vi "Smartwatch - .vi"() -> ()   [LabVIEW 2025]
uses:
  <vilib>/Utility/miscctls.llb/LVPoint32TypeDef.ctl
  <vilib>/Instr/_visa.llb/VISA Configure Serial Port (Instr).vi
panel:
  out "Timer Status":bool
  in  "Smartwatch Display":enum32{"Ekran g³ówny", "Krokomierz", "Stoper"}(tab)
  out "Time Dispay":string
  out "Liczba Kroków (bieg)":i32
  out "Liczba Kroków":i32
  out "Waveform Chart [Magnitude]":cluster{dbl, dbl, dbl}(graph)
  out "Status":string
  in  "STOP Button":bool
  out "Status":bool
  in  "START Button":bool
  in  "Timer START":bool
  in  "Timer STOP":bool
  out "Timer value":u32
  out "Waveform Chart [X+Y+Z]":cluster{dbl, dbl, dbl}(graph)
  out "x*y 3":dbl
  out "x*y 2":dbl
  out "x*y 1":dbl
  out "Smartwatch":picture
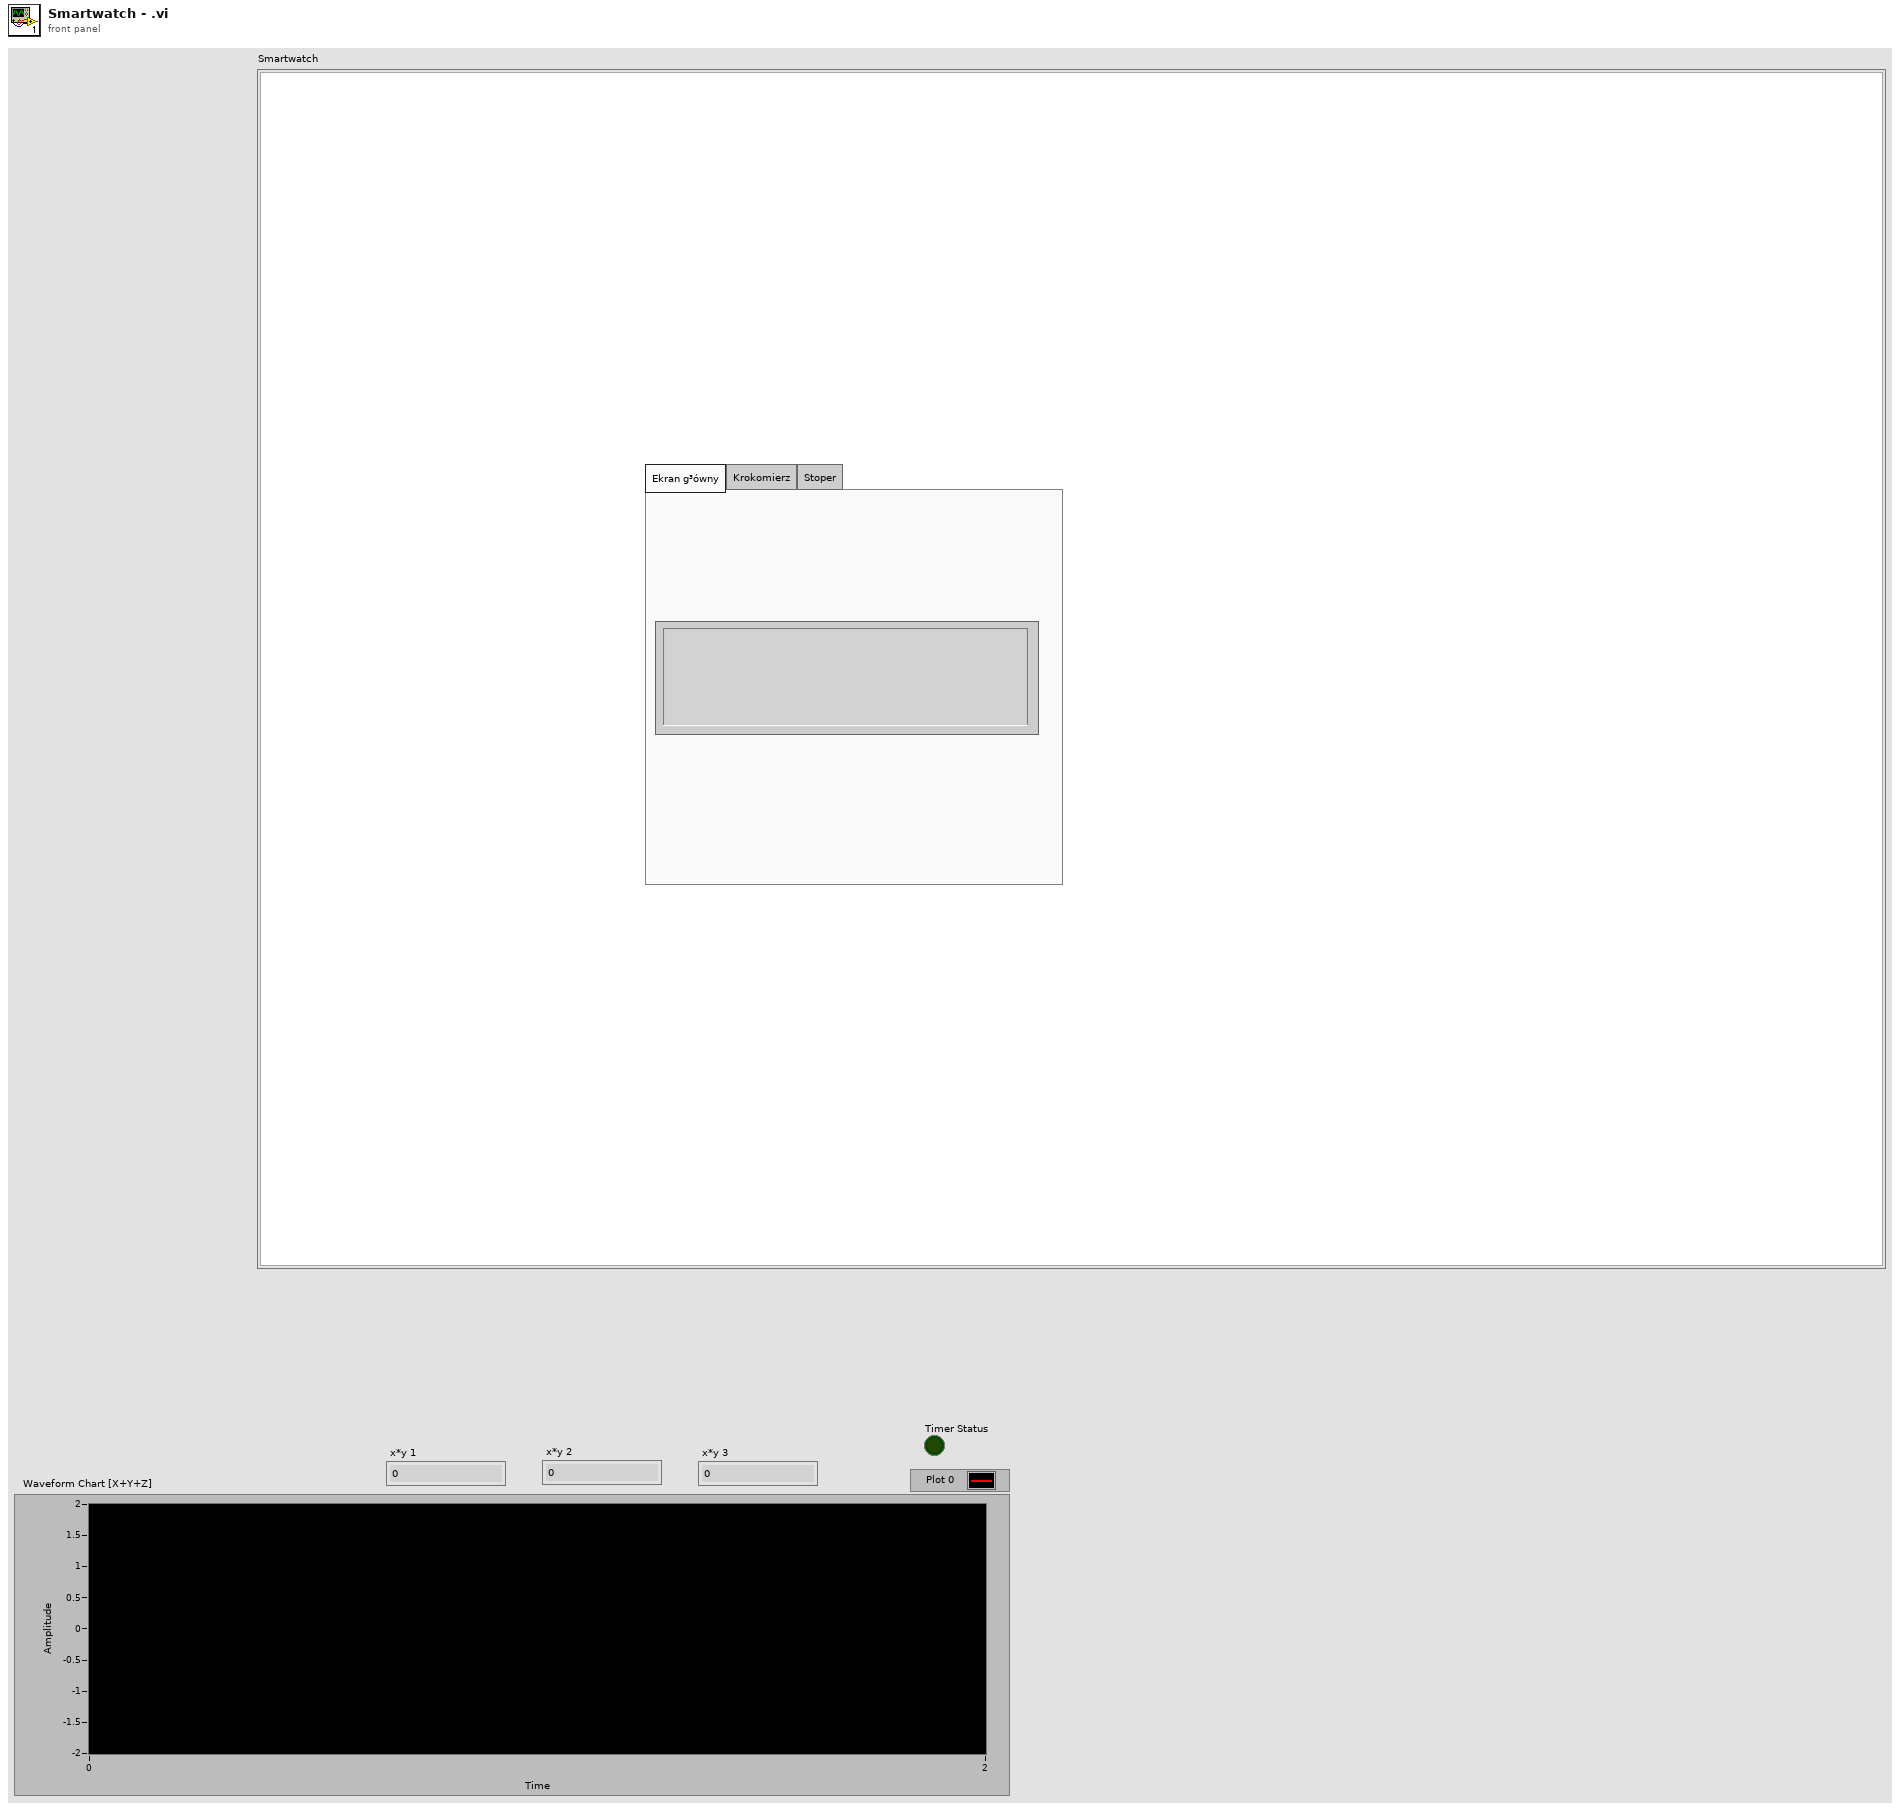
[diagram p1: front panel]
types:
  T1 = typedef "LVPoint32TypeDef.ctl" = cluster{"Horizontal":i32, "Vertical":i32}
  T2 = typedef "imagedata.ctl" = cluster{"image type":i32, "image depth":i32, "image":u8[], "mask":u8[], "colors":u32[], "Rectangle":cluster{"left":i16, "top":i16, "right":i16, "bottom":i16}}
  T3 = cluster{"Acceleration [g] -2.0<->+2.0 ":dbl, "Acceleration [g] -2.0<->+2.0 ":dbl, "Acceleration [g] -2.0<->+2.0 ":dbl}
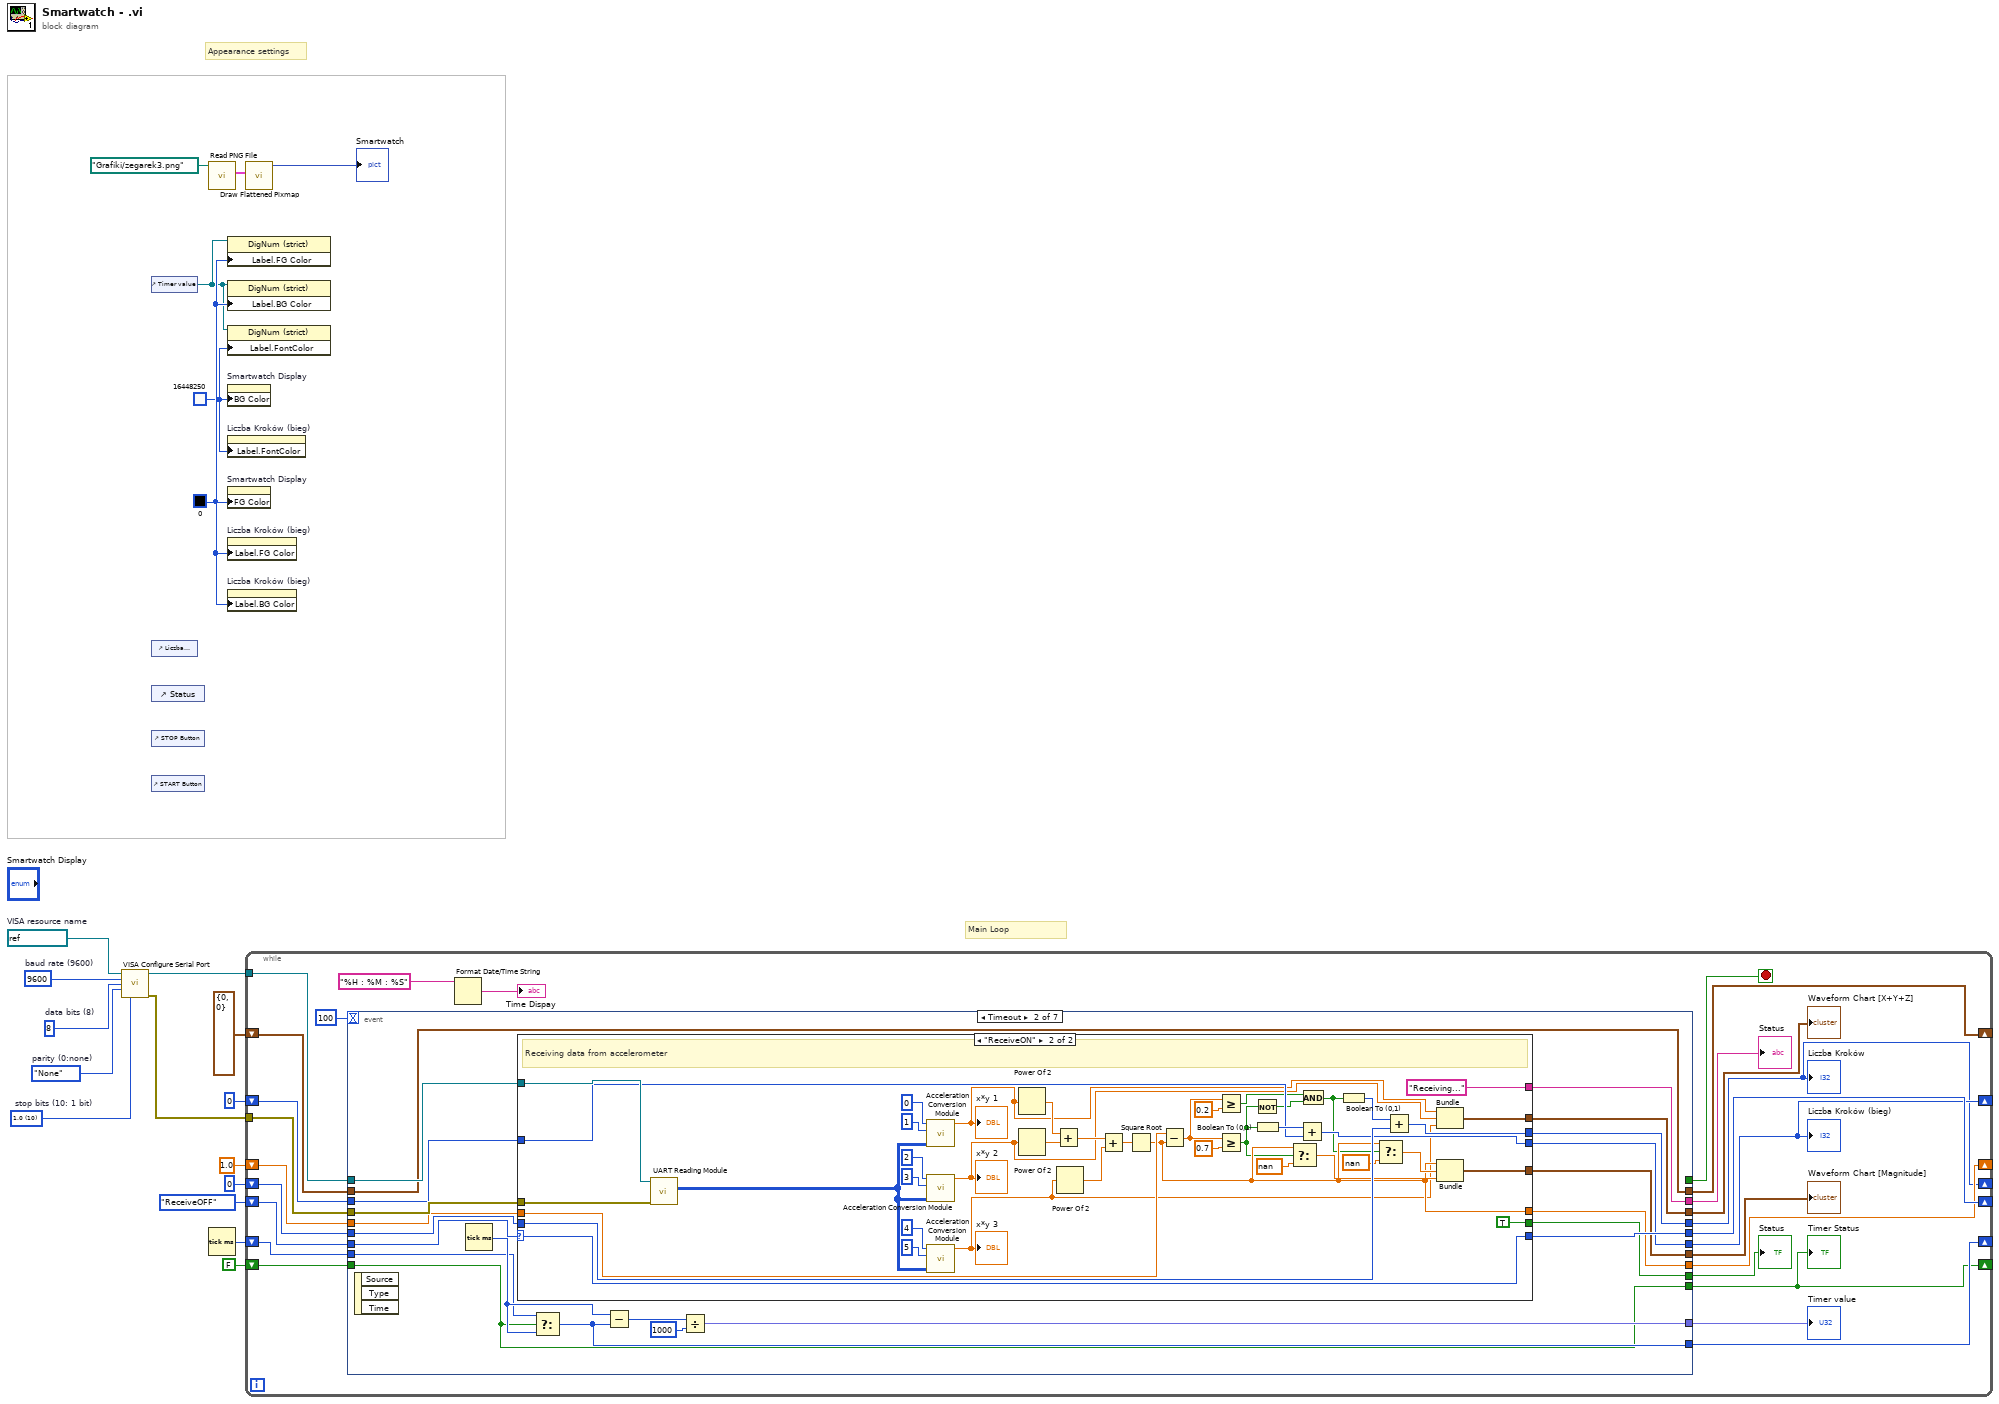
[diagram p0: block diagram]
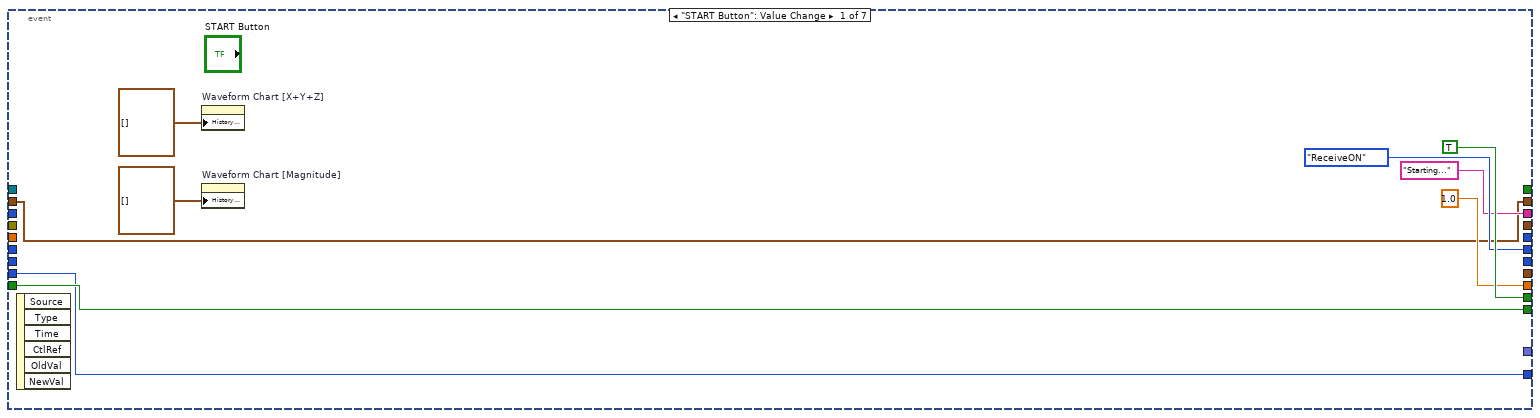
[diagram p2: hidden frame]
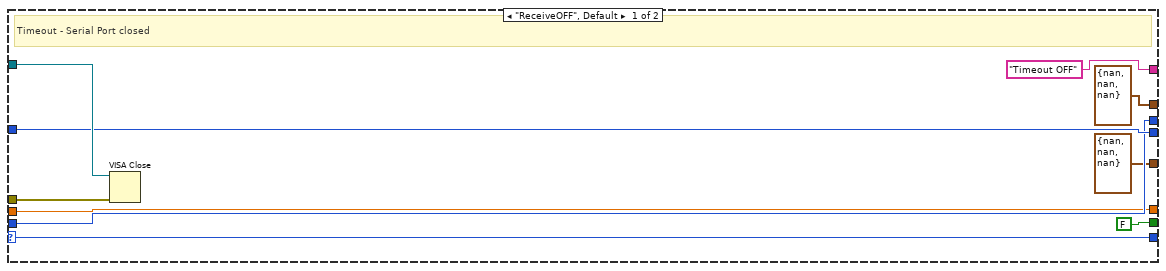
[diagram p3: hidden frame]
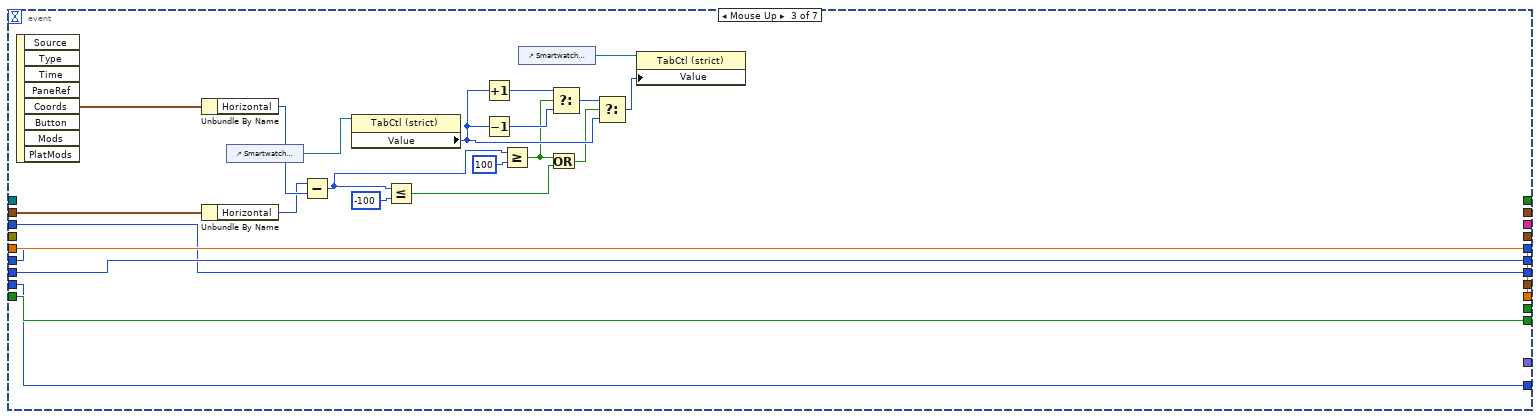
[diagram p4: hidden frame]
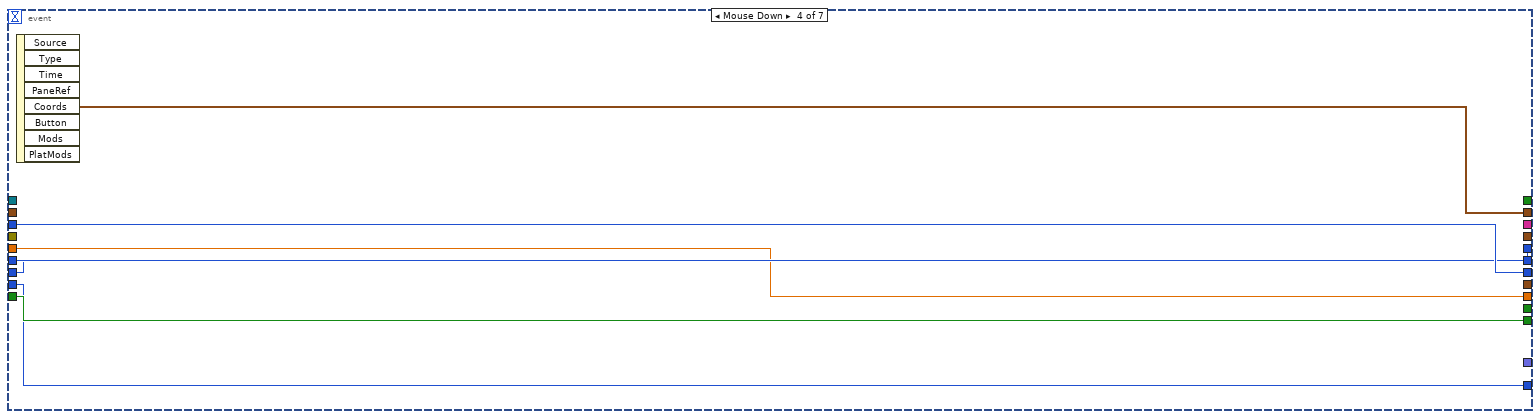
[diagram p5: hidden frame]
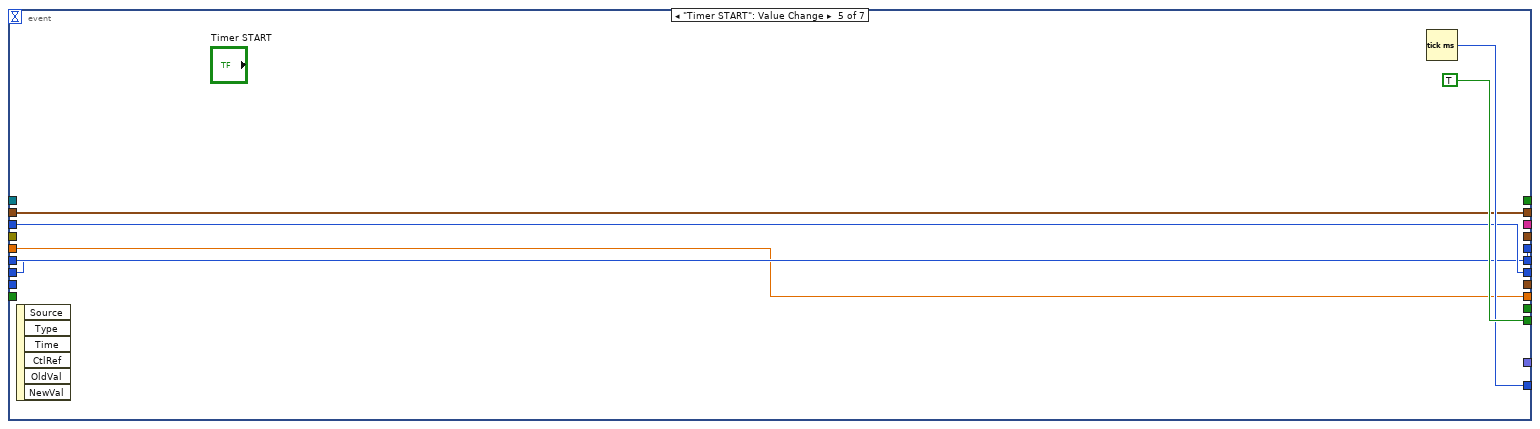
[diagram p6: hidden frame]
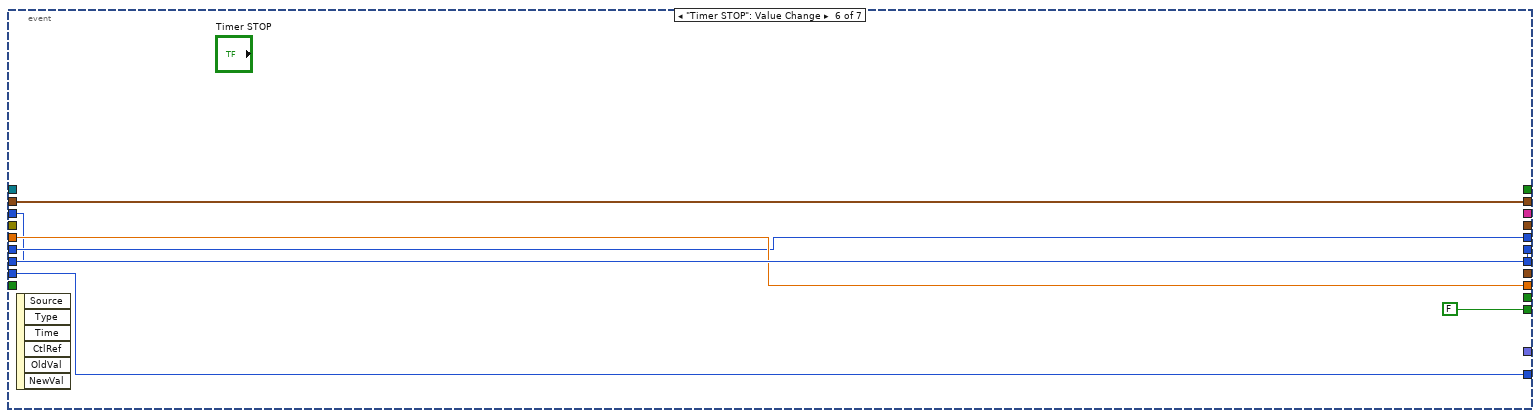
[diagram p7: hidden frame]
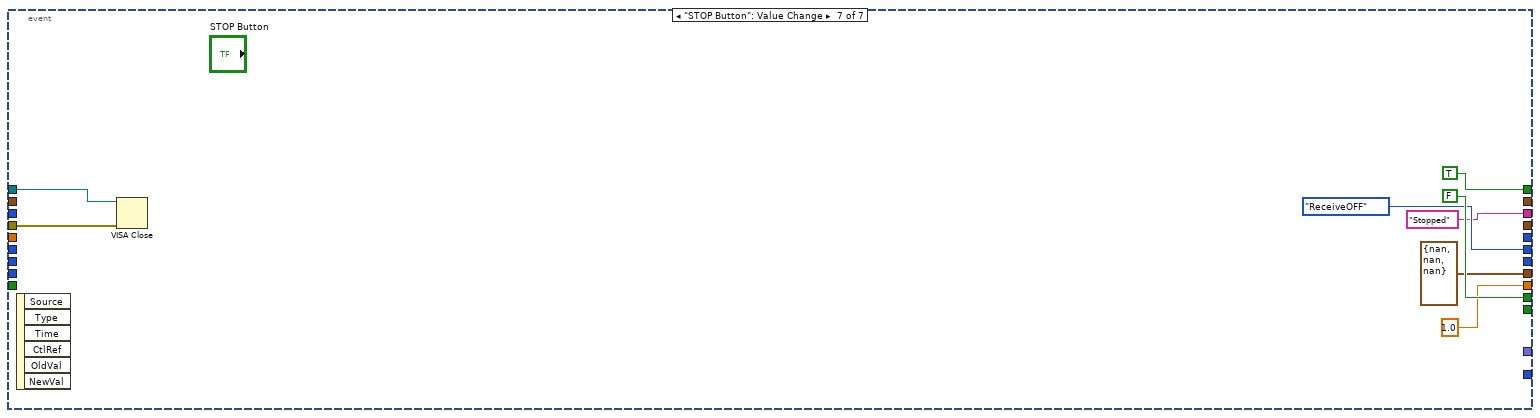
[diagram p8: hidden frame]
diagram:
  w5 = u32 16448250 ("Colors:BG Color")
  w6 = u32 0 ("Colors:BG Color")
  w14 = enum16{"None", "Odd", "Even", "Mark", "Space"}."None"  # parity (0:none)
  w15 = u16 8  # data bits (8)
  w16 = u16 10 items=["1.0"=10, "1.5"=15, "2.0"=20]  # stop bits (10: 1 bit)
  w17 = u32 9600  # baud rate (9600)
  w18 = refnum<visa-resource-name> "COM3"  # VISA resource name
  # "Main Loop"
  # "Appearance settings"
  n1 = call-poly "VISA Configure Serial Port"("VISA resource name"=w18, "baud rate (9600)"=w17, "data bits (8)"=w15, "parity (0:none)"=w14, "stop bits (10: 1 bit)"=w16) -> ("VISA resource name out"=w20:refnum<visa-resource-name>, "error out"=w19:errorcluster)  [unwired: 9 in]
  n2 = control-ref of="Timer value"() -> (w4:refnum<vi>)
  n3 = control-ref of="Liczba Kroków"() -> ()  [unwired: 1 out]
  n4 = control-ref of="Status"() -> ()  [unwired: 1 out]
  n5 = control-ref of="STOP Button"() -> ()  [unwired: 1 out]
  n6 = control-ref of="START Button"() -> ()  [unwired: 1 out]
  n7 = call <vilib>:"Read PNG File.vi"("path to PNG file"=path "Grafiki/zegarek3.png") -> ("image data"=w8:T2)  [unwired: 8 in, 2 out]
  n8 = Tick Count (ms)() -> (millisecond timer value=w3:u32)
  n9 = property on="Property Node" class="DigNum (strict)"(reference=w4, "Label.FG Color"=w6) -> ()  [unwired: 1 in, 2 out]
  n10 = property on="Property Node" class="DigNum (strict)"(reference=w4, "Label.BG Color"=w6) -> ()  [unwired: 1 in, 2 out]
  n11 = property on="Property Node" class="DigNum (strict)"(reference=w4, "Label.FontColor"=w5) -> ()  [unwired: 1 in, 2 out]
  n12 = property on="Smartwatch Display" class="TabCtl (strict)"("BG Color"=w5) -> ()  [unwired: 2 in, 2 out]
  n13 = property on="Liczba Kroków (bieg)" class="DigNum (strict)"("Label.FontColor"=w5) -> ()  [unwired: 2 in, 2 out]
  n14 = property on="Smartwatch Display" class="TabCtl (strict)"("FG Color"=w6) -> ()  [unwired: 2 in, 2 out]
  n15 = property on="Liczba Kroków (bieg)" class="DigNum (strict)"("Label.FG Color"=w6) -> ()  [unwired: 2 in, 2 out]
  n16 = property on="Liczba Kroków (bieg)" class="DigNum (strict)"("Label.BG Color"=w6) -> ()  [unwired: 2 in, 2 out]
  n17 = call <vilib>:"Draw Flattened Pixmap.vi"("image data"=w8) -> ("new picture"=→"Smartwatch":picture)  [unwired: 8 in]
  n18 = while {
    tunnel: w19 -> [w44]
    tunnel: w20 -> [w45]
    shift-right: [w40] -> _
    shift-left: enum16{"ReceiveOFF", "ReceiveON"}."ReceiveOFF" -> [w41]
    shift-right: [w37] -> _
    shift-left: 1.0 -> [w36]
    shift-right: [w32] -> _
    shift-left: 0 -> [w35]
    shift-right: [w33] -> _
    shift-left: 0 -> [w34]
    shift-right: [w29] -> _
    shift-left: w3 -> [w25]
    shift-right: [w26] -> _
    shift-left: FALSE -> [w28]
    shift-right: [w23] -> _
    shift-left: T1 {"Horizontal"=0, "Vertical"=0} ("Coords") -> [w24]
    stop <- w42 stop-if-true
    n19 = event shown="[1] Timeout" {
      selector: _ -> [_ _ _ _ _ _ _]
      dyn-events: _ -> [_ _ _ _ _ _ _]
      timeout: 100 -> [_ _ _ _ _ _ _]
      tunnel: w45 -> [_ w74 _ _ _ _ w179]
      tunnel: w44 -> [_ w73 _ _ _ _ w178]
      tunnel: [TRUE w72 _ _ _ _ FALSE] -> w43
      tunnel: [_ _ _ _ _ _ TRUE] -> w42
      tunnel: w41 -> [_ w76 w133 w153 w159 w168 _]
      tunnel: [enum16{"ReceiveOFF", "ReceiveON"}."ReceiveON" w75 w133 w153 w159 w168 enum16{"ReceiveOFF", "ReceiveON"}."ReceiveOFF"] -> w40
      tunnel: ["Starting..." ("Status") w71 _ _ _ _ "Stopped" ("Status")] -> w38
      tunnel: [1.0 ("Magnitude Old") w70 w132 w154 w160 w167 1.0] -> w37
      tunnel: w36 -> [_ w69 w132 w154 w160 w167 _]
      tunnel: w35 -> [_ w68 w130 w155 w161 w166 _]
      tunnel: w34 -> [_ w67 w131 w156 w162 w165 _]
      tunnel: [_ w66 w130 w155 w161 w166 _] -> w32
      tunnel: [_ w65 w131 w156 w162 w165 _] -> w33
      tunnel: [_ w64 _ _ _ _ cluster{dbl, dbl, dbl} {nan, nan, nan}] -> w31
      tunnel: [_ w63 _ _ _ _ _] -> w30
      tunnel: w28 -> [w47 w56 w129 w152 _ _ _]
      tunnel: w25 -> [w46 w60 w128 w151 _ w169 _]
      tunnel: [w46 w58 w128 w151 w163 w169 _] -> w29
      tunnel: [_ w57 _ _ _ _ _] -> w27
      tunnel: [w47 w56 w129 w152 TRUE FALSE _] -> w26
      tunnel: w24 -> [w48 w55 w136 _ w158 w170 _]
      tunnel: [w48 w55 _ w157 w158 w170 _] -> w23
      event "START Button": Value Change {
        n20 = event-data() -> ()  [unwired: 1 in, 6 out]
        n21 = property on="Waveform Chart [X+Y+Z]" class="WFChart (strict)"("History Data"=cluster{dbl, dbl, dbl}[] []) -> ()  [unwired: 2 in, 2 out]
        n22 = property on="Waveform Chart [Magnitude]" class="WFChart (strict)"("History Data"=cluster{dbl, dbl, dbl}[] []) -> ()  [unwired: 2 in, 2 out]
      }
      event Timeout {
        n23 = event-data() -> ()  [unwired: 1 in, 3 out]
        n24 = Tick Count (ms)() -> (millisecond timer value=w62:u32)
        n25 = case shown="\"ReceiveON\"" w76 {
          selector: w76 -> [w78 w99]
          tunnel: [w78 w99] -> w75
          tunnel: w74 -> [w86 w127]
          tunnel: w73 -> [w85 w126]
          tunnel: [FALSE TRUE] -> w72
          tunnel: ["Timeout OFF" ("Status") "Receiving..." ("Status")] -> w71
          tunnel: [w80 w98] -> w70
          tunnel: w69 -> [w80 w114]
          tunnel: w68 -> [w81 w108]
          tunnel: w67 -> [w82 w109]
          tunnel: [w81 w106] -> w66
          tunnel: [w82 w105] -> w65
          tunnel: [cluster{dbl, dbl, dbl} {nan, nan, nan} w100] -> w64
          tunnel: [cluster{dbl, dbl, dbl} {nan, nan, nan} w90] -> w63
          frame "ReceiveOFF", Default {
            # "Timeout - Serial Port closed"
            n26 = VISA Close(VISA resource name=w86, error in (no error)=w85) -> ()  [unwired: 1 out]
          }
          frame "ReceiveON" {
            # "Receiving data from accelerometer"
            n27 = call "UART Reading Module.vi"("error in (no error)"=w126, "VISA Refnum in"=w127) -> ("Array with 6 col"=w121:u8[][])  [unwired: 7 in, 2 out]
            n28 = call "Acceleration Conversion Module.vi"("Array Input (1 row 6 col)"=w121, "Second column"=1, "First column"=0) -> ("Acceleration [g] -2.0<->+2.0"=w89:dbl)  [unwired: 6 in]
            "x*y 1" <- w89
            n29 = call "Acceleration Conversion Module.vi"("Array Input (1 row 6 col)"=w121, "Second column"=3, "First column"=2) -> ("Acceleration [g] -2.0<->+2.0"=w88:dbl)  [unwired: 6 in]
            "x*y 2" <- w88
            n30 = call "Acceleration Conversion Module.vi"("Array Input (1 row 6 col)"=w121, "Second column"=5, "First column"=4) -> ("Acceleration [g] -2.0<->+2.0"=w87:dbl)  [unwired: 6 in]
            "x*y 3" <- w87
            n31 = Power Of 2(x=w89) -> (2^x=w93:dbl)
            n32 = Power Of 2(x=w88) -> (2^x=w92:dbl)
            n33 = Add(x=w93, y=w92) -> (x+y=w116:dbl)
            n34 = Power Of 2(x=w87) -> (2^x=w91:dbl)
            n35 = Add(x=w116, y=w91) -> (x+y=w115:dbl)
            n36 = Square Root(x=w115) -> (sqrt(x)=w98:dbl)
            n37 = Subtract(x=w114, y=w98) -> (x-y=w112:dbl)
            n38 = Greater Or Equal?(x=w112, y=0.2) -> (x >= y?=w102:bool)
            n39 = Greater Or Equal?(x=w112, y=0.7) -> (x >= y?=w95:bool)
            n40 = Not(x=w95) -> (.not. x?=w104:bool)
            n41 = Boolean To (0,1)(Boolean=w95) -> (0, 1=w110:i16)
            n42 = Select(t=w98, s=w95, f=nan) -> (s? t:f=w97:dbl)
            n43 = Add(x=w110, y=w109) -> (x+y=w105:i32)
            n44 = And(x=w102, y=w104) -> (x .and. y?=w94:bool)
            n45 = Boolean To (0,1)(Boolean=w94) -> (0, 1=w107:i16)
            n46 = Select(t=w98, s=w94, f=nan) -> (s? t:f=w101:dbl)
            n47 = Add(x=w107, y=w108) -> (x+y=w106:i32)
            n48 = Bundle("Acceleration [g] -2.0<->+2.0"=w89, "Acceleration [g] -2.0<->+2.0"=w88, "Acceleration [g] -2.0<->+2.0"=w87) -> (w90:T3)  [unwired: 1 in]
            n49 = Bundle(w98, w101, w97) -> (w100:cluster{dbl, dbl, dbl})  [unwired: 1 in]
          }
        }
        n50 = Select(t=w60, s=w56, f=w62) -> (s? t:f=w58:u32)
        n51 = Subtract(x=w62, y=w58) -> (x-y=w61:u32)
        n52 = Divide(x=w61, y=u32 1000) -> (x/y=w57:fxp<+,32,16>)
      }
      event Mouse Up {
        n53 = event-data() -> ("Coords"=w137:T1)  [unwired: 1 in, 7 out]
        n54 = Unbundle By Name(w137) -> ("Horizontal"=w150:i32)
        n55 = Unbundle By Name(w136) -> ("Horizontal"=w149:i32)
        n56 = control-ref of="Smartwatch Display"() -> (w135:refnum<vi>)
        n57 = Subtract(x=w149, y=w150) -> (x-y=w146:i32)
        n58 = property on="Property Node" class="TabCtl (strict)"(reference=w135) -> ("Value"=w142:enum32{"Ekran g³ówny", "Krokomierz", "Stoper"})  [unwired: 1 in, 2 out]
        n59 = Less Or Equal?(x=w146, y=-100) -> (x <= y?=w140:bool)
        n60 = Increment(x=w142) -> (x+1=w145:enum32{"Ekran g³ówny", "Krokomierz", "Stoper"})
        n61 = Decrement(x=w142) -> (x-1=w144:enum32{"Ekran g³ówny", "Krokomierz", "Stoper"})
        n62 = Greater Or Equal?(x=w146, y=100) -> (x >= y?=w141:bool)
        n63 = control-ref of="Smartwatch Display"() -> (w134:refnum<vi>)
        n64 = Or(x=w141, y=w140) -> (x .or. y?=w139:bool)
        n65 = Select(t=w145, s=w141, f=w144) -> (s? t:f=w143:enum32{"Ekran g³ówny", "Krokomierz", "Stoper"})
        n66 = Select(t=w143, s=w139, f=w142) -> (s? t:f=w138:enum32{"Ekran g³ówny", "Krokomierz", "Stoper"})
        n67 = property on="Property Node" class="TabCtl (strict)"(reference=w134, "Value"=w138) -> ()  [unwired: 1 in, 2 out]
      }
      event Mouse Down {
        n68 = event-data() -> ("Coords"=w157:T1)  [unwired: 1 in, 7 out]
      }
      event "Timer START": Value Change {
        n69 = event-data() -> ()  [unwired: 1 in, 6 out]
        n70 = Tick Count (ms)() -> (millisecond timer value=w163:u32)
      }
      event "Timer STOP": Value Change {
        n71 = event-data() -> ()  [unwired: 1 in, 6 out]
      }
      event "STOP Button": Value Change {
        n72 = event-data() -> ()  [unwired: 1 in, 6 out]
        n73 = VISA Close(VISA resource name=w179, error in (no error)=w178) -> ()  [unwired: 1 out]
      }
    }
    "Status" <- w43
    "Status" <- w38
    "Liczba Kroków (bieg)" <- w33
    "Liczba Kroków" <- w32
    "Waveform Chart [Magnitude]" <- w31
    "Waveform Chart [X+Y+Z]" <- w30
    "Timer value" <- w27
    "Timer Status" <- w26
    n74 = Format Date/Time String(time format string (%c)="%H : %M : %S") -> (date/time string=→"Time Dispay":string)  [unwired: 2 in]
  }
